vi "5. NumericOps3.vi"() -> ()   [LabVIEW 2019]
panel:
  out "Speed of Light":ext[unit]=299792458.0
  out "Planks Constant":ext[unit]=6.62607004e-34
  out "exp":dbl=2.718281828459045
  out "Pi":dbl=3.141592653589793
  out "x*y":dbl
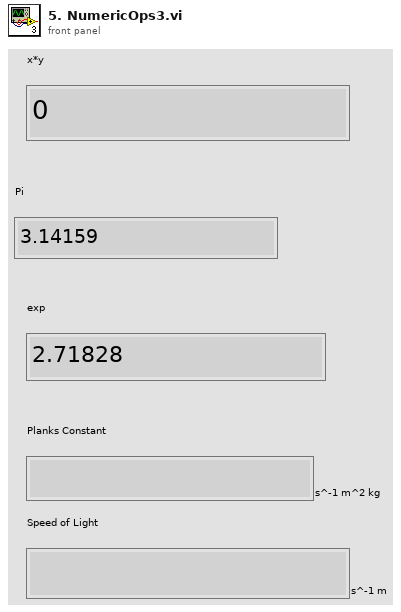
[diagram p1: front panel]
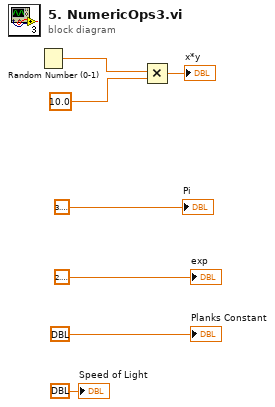
[diagram p0: block diagram]
diagram:
  n1 = Random Number (0-1)() -> (number: 0 to 1=w7:dbl)
  n2 = Multiply(x=w7, y=10.0) -> (x*y=→"x*y":dbl)
  "Pi" <- 3.141592653589793
  "exp" <- 2.718281828459045
  "Planks Constant" <- ext[unit] 6.62607004e-34
  "Speed of Light" <- ext[unit] 299792458.0
